vi "Digital Pattern Wrap Around.vi"(9 "Rotations":u16, 11 "x":dbl) -> (3 "x":dbl)   [LabVIEW 2015, in "Engine Simulation Toolkit System Explorer.lvlib"]
uses:
  Engine Simulation Toolkit System Explorer.lvlib
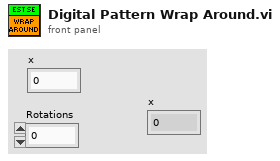
[diagram p1: front panel]
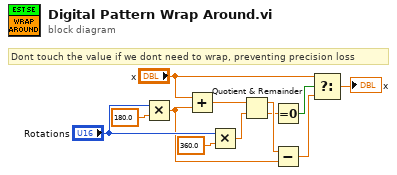
[diagram p0: block diagram]
diagram:
  # "Dont touch the value if we dont need to wrap, preventing precision loss"
  n1 = Multiply(x="Rotations", y=180.0 ("t")) -> (x*y=w6:dbl)
  n2 = Add(x="x", y=w6) -> (x+y=w12:dbl)
  n3 = Multiply(x="Rotations", y=360.0 ("t")) -> (x*y=w9:dbl)
  n4 = Quotient & Remainder(x=w12, y=w9) -> (x-y*floor(x/y)=w11:dbl, floor(x/y)=w5:dbl)
  n5 = Equal To 0?(x=w5) -> (x = 0?=w4:bool)
  n6 = Subtract(x=w11, y=w6) -> (x-y=w2:dbl)
  n7 = Select(t="x", s=w4, f=w2) -> (s? t:f=→"x":dbl)
